vi "SaveConfig.vi"(8 "error in (no error)":errorcluster, 11 "GRMActor in":refnum<class "DataLoggerUI.lvclass">) -> (0 "error out":errorcluster, 3 "GRMActor out":refnum<class "DataLoggerUI.lvclass">)   [LabVIEW 2020, in "DataLogger.lvlib" / "DataLoggerUI.lvlib" / "DataLoggerUI.lvclass"]
uses:
  DataLoggerUI.lvclass
  DataLoggerUI.lvclass/DataLoggerUI.ctl
  Hardware Abstraction Layer/Component/GenericActor/GenericActor/GenericController.lvclass
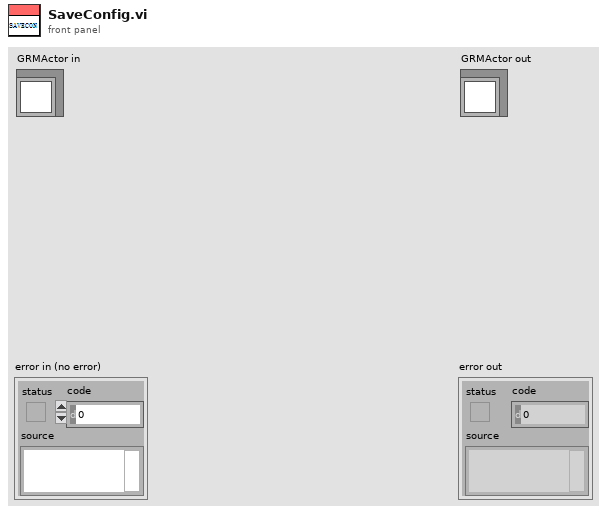
[diagram p1: front panel]
types:
  T1 = typedef "NI_LVConfig.lvlib/Config Data RefNum.ctl" = refnum<k1>
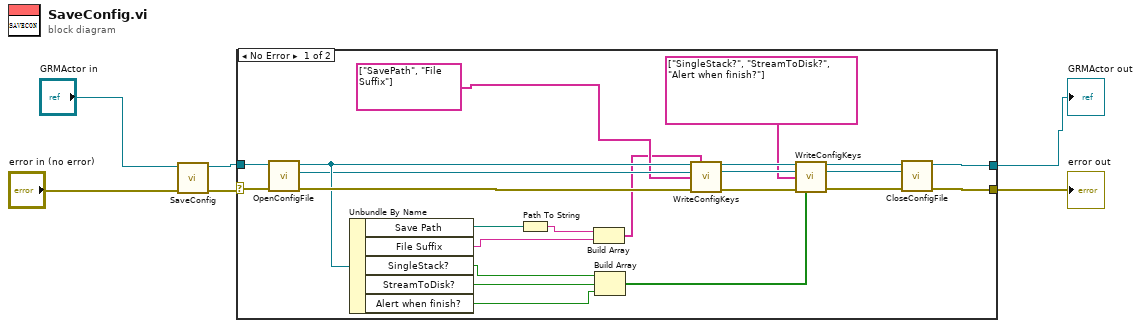
[diagram p0: block diagram]
diagram:
  n1 = call-parent "SaveConfig.vi"("error in (no error)"="error in (no error)", "GRMActor in"="GRMActor in") -> ("error out"=w4:errorcluster, "GRMActor out"=w3:refnum<class "DataLoggerUI.lvclass">)  [unwired: 8 in]
  n2 = case shown="No Error" w4 {
    selector: w4 -> [w29 w30]
    tunnel: [w26 w30] -> w1
    tunnel: [w25 w31] -> w2
    tunnel: w3 -> [w24 w31]
    frame No Error {
      n3 = call-dynamic "OpenConfigFile.vi"("error in (no error)"=w29, "GRMActor in"=w24) -> ("error out"=w27:errorcluster, "refnum"=w22:T1, "GRMActor out"=w23:refnum<class "DataLoggerUI.lvclass">)  [unwired: 7 in]
      n4 = Unbundle By Name(w23) -> ("Save Path"=w9:path, "File Suffix"=w8:string, "SingleStack?"=w21:bool, "StreamToDisk?"=w20:bool, "Alert when finish?"=w19:bool)
      n5 = Path To String(path=w9) -> (string=w10:string)
      n6 = Build Array(w10, w8) -> (w7:string[])
      n7 = Build Array(w21, w20, w19) -> (w11:bool[])
      n8 = call-dynamic "WriteConfigKeys.vi"("GRMActor in"=w23, "StringValues"=w7, "Config Refnum"=w22, "Keys"=string[] ["SavePath", "File Suffix"] ("Values"), "error in (no error)"=w27) -> ("GRMActor out"=w17:refnum<class "DataLoggerUI.lvclass">, "Config Refnum dup"=w15:T1, "error out"=w28:errorcluster)  [unwired: 8 in]
      n9 = call-dynamic "WriteConfigKeys.vi"("GRMActor in"=w17, "Config Refnum"=w15, "Keys"=string[] ["SingleStack?", "StreamToDisk?", "Alert when finish?"], "error in (no error)"=w28, "BoolValues"=w11) -> ("GRMActor out"=w16:refnum<class "DataLoggerUI.lvclass">, "Config Refnum dup"=w14:T1, "error out"=w18:errorcluster)  [unwired: 8 in]
      n10 = call-dynamic "CloseConfigFile.vi"("error in (no error)"=w18, "refnum"=w14, "GRMActor in"=w16) -> ("error out"=w26:errorcluster, "GRMActor out"=w25:refnum<class "DataLoggerUI.lvclass">)  [unwired: 7 in]
    }
    frame Error {
    }
  }
  "error out" <- w1
  "GRMActor out" <- w2
